vi "Lockin.DAQ.Write AO.vi"(8 "error in (no error)":errorcluster, 10 "AO []":waveform(dbl)[](array[waveform]), 11 "Lockin.DAQ in":refnum<class "Lockin.DAQ.lvclass">) -> (0 "error out":errorcluster, 1 "AO time (ms)":u32=53, 3 "Lockin.DAQ out":refnum<class "Lockin.DAQ.lvclass">)   [LabVIEW 2016, in "Lockin.DAQ.lvclass"]
uses:
  Lockin.DAQ.lvclass
  Lockin.DAQ.lvclass/Lockin.DAQ.ctl
  <vilib>/DAQmx/write.llb/DAQmx Write (Analog 1D Wfm NChan NSamp).vi
  <vilib>/DAQmx/miscellaneous.llb/DAQmx Fill In Error Info.vi
panel:
  out "P Check":bool[](array[boolean])
  out "# samples written":u32[](array[numeric])
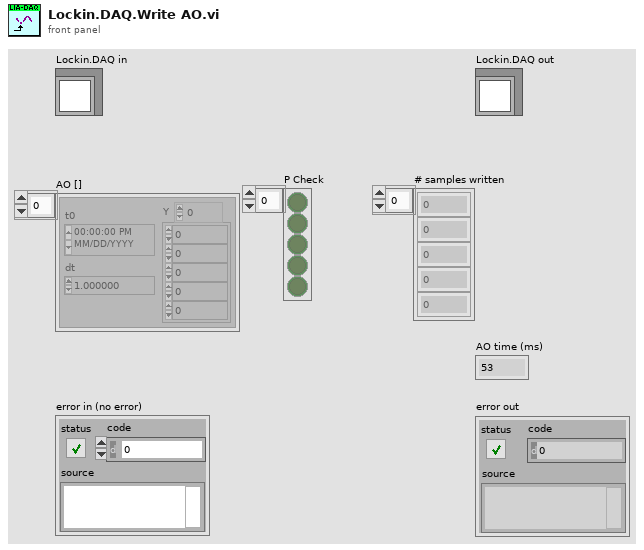
[diagram p1: front panel]
types:
  T1 = enum16{"static", "dynamic", "dynamic asynchronous"}
  T2 = typedef "Lockin.DAQ.lvclass/DAQType-enum.ctl" = enum16{"None", "USB 4431", "PXI 446x"}
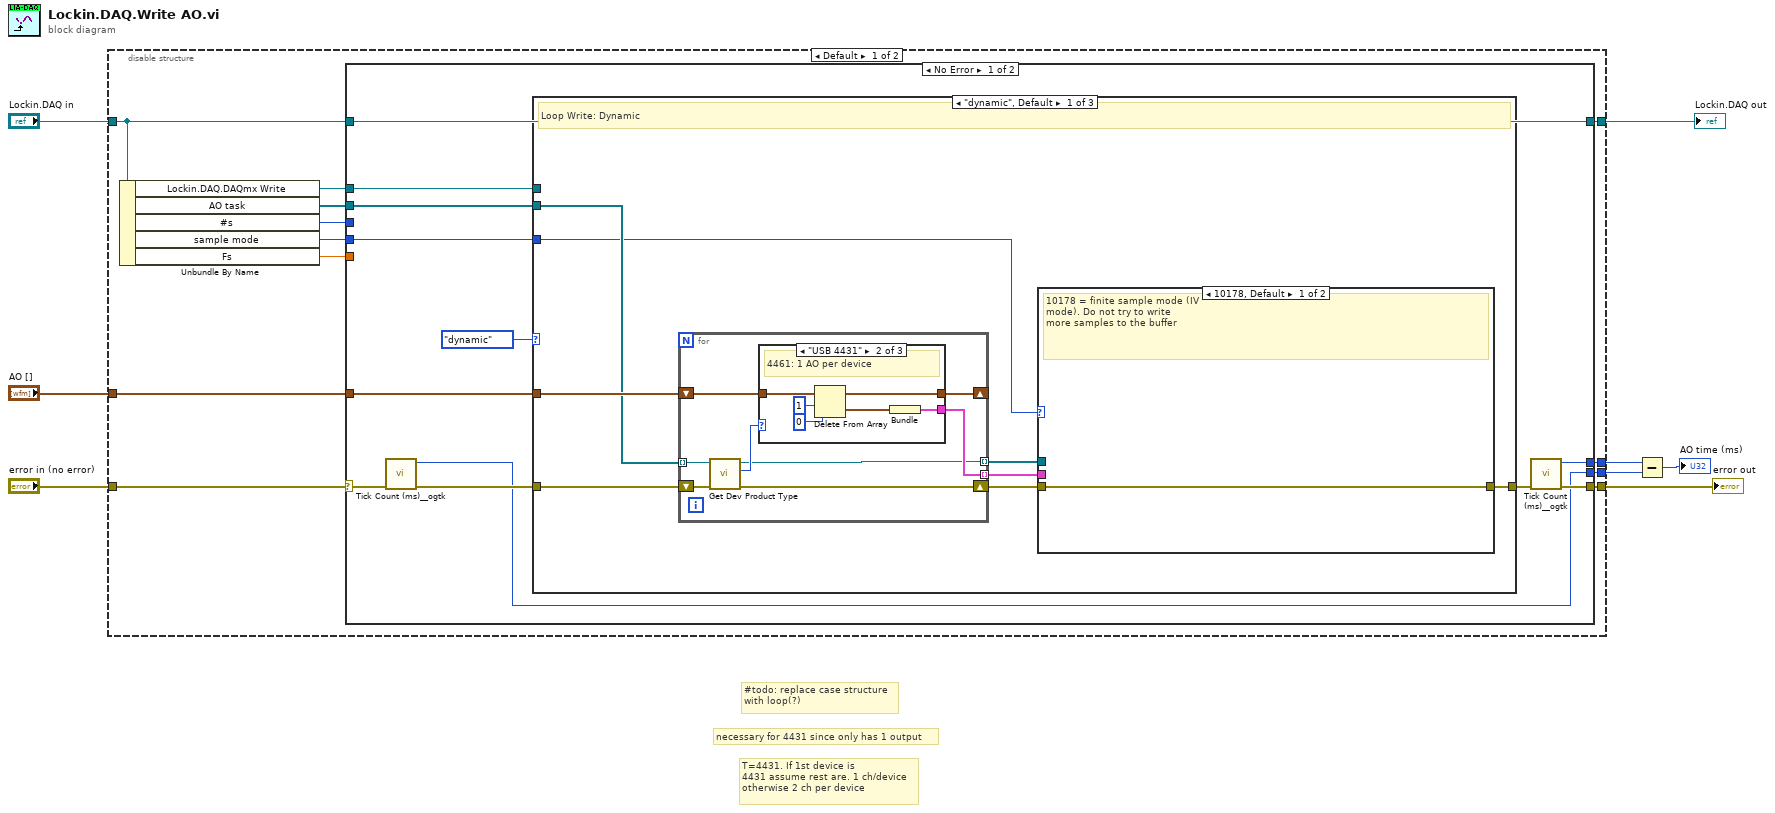
[diagram p0: block diagram]
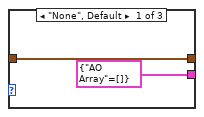
[diagram p2: hidden frame]
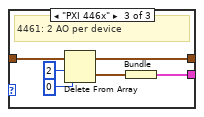
[diagram p3: hidden frame]
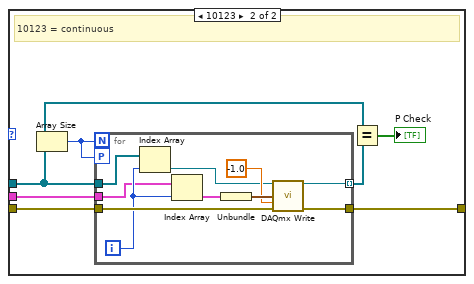
[diagram p4: hidden frame]
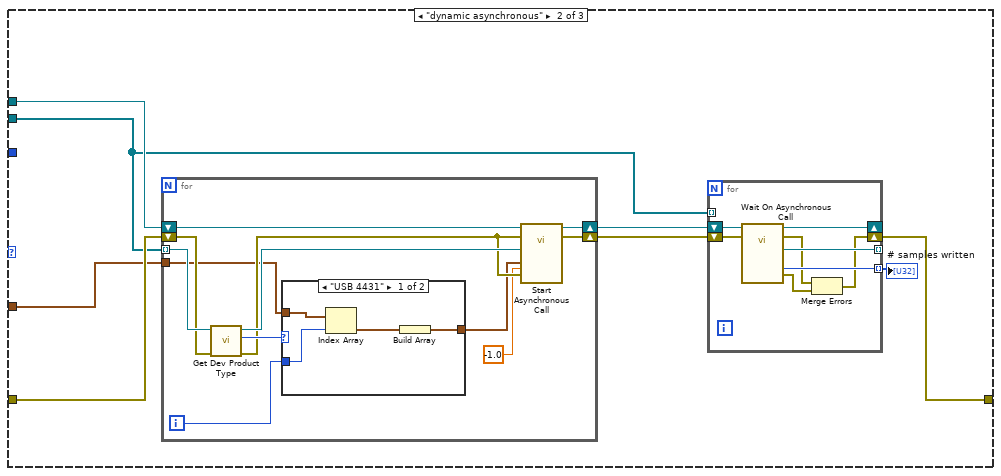
[diagram p5: hidden frame]
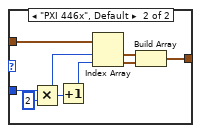
[diagram p6: hidden frame]
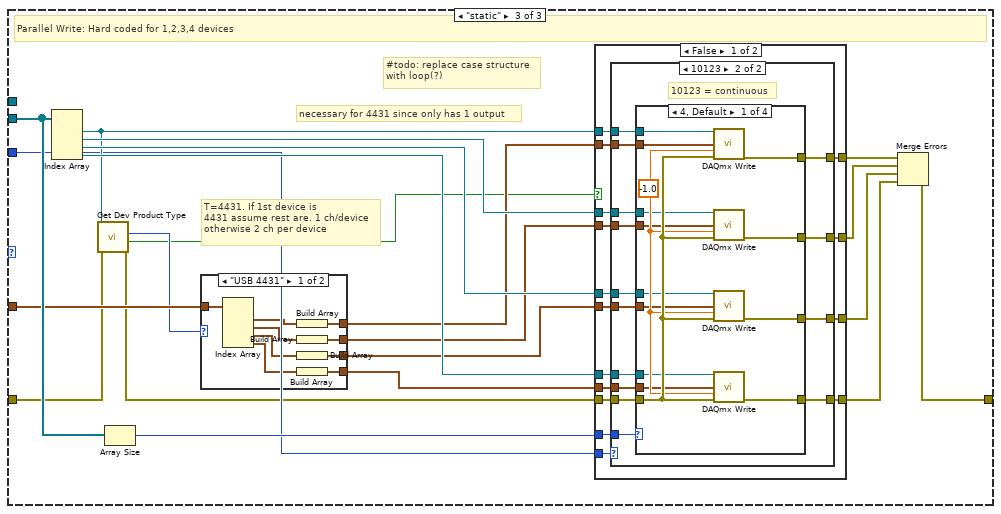
[diagram p7: hidden frame]
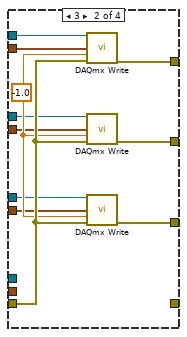
[diagram p9: hidden frame]
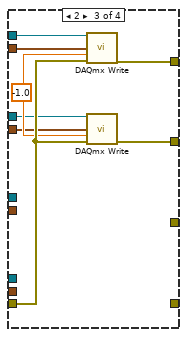
[diagram p10: hidden frame]
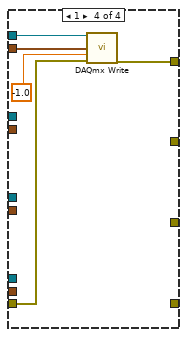
[diagram p11: hidden frame]
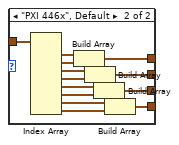
[diagram p13: hidden frame]
diagram:
  # "#todo: replace case structure\nwith loop(?)"
  # "T=4431. If 1st device is \n4431 assume rest are. 1 ch/device\notherwise 2 ch per device"
  # "necessary for 4431 since only has 1 output"
  n1 = disable-structure shown="Default" {
    disable-tunnel: [w18 w236] -> w3
    disable-tunnel: "Lockin.DAQ in" -> [w16 _]
    disable-tunnel: "AO []" -> [w17 w235]
    disable-tunnel: "error in (no error)" -> [w10 w236]
    disable-tunnel: [w15 _] -> w2
    disable-tunnel: [w14 _] -> w7
    disable-tunnel: [w13 _] -> w6
    frame condition #0 (active) {
      n2 = Unbundle By Name(w16) -> ("Lockin.DAQ.DAQmx Write"=w9:refnum<vi>, "AO task"=w11:refnum<k21>[], "#s"=w20:i32, "sample mode"=w19:i32, "Fs"=w12:dbl)
      n3 = case shown="No Error" w10 {
        selector: w10 -> [w25 w233]
        tunnel: w20 -> [_ _]
        tunnel: w19 -> [w26 _]
        tunnel: [w29 w233] -> w18
        tunnel: w17 -> [w31 _]
        tunnel: w11 -> [w32 _]
        tunnel: w16 -> [w27 w234]
        tunnel: [w27 w234] -> w15
        tunnel: [w28 _] -> w14
        tunnel: [w21 _] -> w13
        tunnel: w12 -> [_ _]
        tunnel: w9 -> [w23 _]
        frame No Error {
          n4 = call <userlib>:"Tick Count (ms)__ogtk.vi"("error in (no error)"=w25) -> ("error out"=w24:errorcluster, "millisecond timer value"=w21:u32)  [unwired: 9 in]
          n5 = case shown="\"dynamic\", Default" T1."dynamic" ("Enum") {
            tunnel: w32 -> [w35 w82 w141]
            tunnel: w31 -> [w38 w84 w140]
            tunnel: [w37 w83 w139] -> w30
            tunnel: w26 -> [w33 _ w125]
            tunnel: w24 -> [w40 w86 w123]
            tunnel: w23 -> [_ w85 _]
            frame "dynamic", Default {
              # "Loop Write: Dynamic"
              n6 = for {
                tunnel: [w44] -> w36 mode=indexing
                shift-right: [w47] -> w39
                shift-left: w40 -> [w48]
                tunnel: w35 -> [w43] mode=indexing
                tunnel: [w42] -> w34 mode=indexing
                shift-right: [w41] -> _
                shift-left: w38 -> [w46]
                n7 = call "Get Dev Product Type.vi"("error in (no error)"=w48, "Refnum in"=w43) -> ("error out"=w47:errorcluster, "DAQ Type"=w45:T2, "Refnum out"=w42:refnum<k21>)  [unwired: 6 in, 1 out]
                n8 = case shown="\"USB 4431\"" w45 {
                  tunnel: w46 -> [w50 w56 w62]
                  tunnel: [w50 w55 w61] -> w41
                  tunnel: [cluster{"AO Array":waveform(dbl)[]} {"AO Array"=[]} w53 w58] -> w44
                  frame "None", Default {
                  }
                  frame "USB 4431" {
                    # "4461: 1 AO per device"
                    n9 = Delete From Array(array=w56, length=1, index=0) -> (deleted portion=w52:waveform(dbl)[], array with subset deleted=w55:waveform(dbl)[])
                    n10 = Bundle("AO []"=w52) -> (w53:cluster{"AO []":waveform(dbl)[]})  [unwired: 1 in]
                  }
                  frame "PXI 446x" {
                    # "4461: 2 AO per device"
                    n11 = Delete From Array(array=w62, length=2, index=0) -> (deleted portion=w59:waveform(dbl)[], array with subset deleted=w61:waveform(dbl)[])
                    n12 = Bundle("AO []"=w59) -> (w58:cluster{"AO []":waveform(dbl)[]})  [unwired: 1 in]
                  }
                }
              }
              n13 = case shown="10178, Default" w33 {
                tunnel: [w63 w68] -> w37
                tunnel: w34 -> [_ w65]
                tunnel: w36 -> [_ w70]
                tunnel: w39 -> [w63 w69]
                frame 10178, Default {
                  # "10178 = finite sample mode (IV\nmode). Do not try to write\nmore samples to the buffer"
                }
                frame 10123 {
                  # "10123 = continuous"
                  n14 = Array Size(array=w65) -> (size(s)=w67:i32)
                  n15 = for {
                    N: w67 -> [_]
                    tunnel: w65 -> [w71]
                    tunnel: w70 -> [w72]
                    tunnel: w69 -> [w80]
                    tunnel: [w79] -> w68
                    workers-P: w67 -> [_]
                    tunnel: [w76] -> w66 mode=indexing
                    i -> [w73]
                    n16 = Index Array(array=w71, index=w73) -> (element=w74:refnum<k21>)
                    n17 = Index Array(array=w72, index=w73) -> (element=w75:cluster{"AO []":waveform(dbl)[]})
                    n18 = Unbundle(w75) -> ("AO []"=w78:waveform(dbl)[])
                    n19 = call-poly <vilib>:"DAQmx Write.vi"("task/channels in"=w74, "data"=w78, "timeout"=-1.0, "error in"=w80) -> ("task out"=w76:refnum<k21>, "error out"=w79:errorcluster)  [unwired: 9 in, 1 out]
                  }
                  n20 = Equal?(x=w65, y=w66) -> (x = y?=→"P Check":bool[])
                }
              }
            }
            frame "dynamic asynchronous" {
              n21 = for {
                shift-right: [w100] -> w87
                shift-left: w86 -> [w94]
                shift-right: [w99] -> w88
                shift-left: w85 -> [w98]
                tunnel: w82 -> [w96] mode=indexing
                tunnel: w84 -> [w92]
                i -> [w91]
                n22 = call "Get Dev Product Type.vi"("error in (no error)"=w94, "Refnum in"=w96) -> ("error out"=w93:errorcluster, "DAQ Type"=w97:T2, "Refnum out"=w95:refnum<k21>)  [unwired: 6 in, 1 out]
                n23 = case shown="\"USB 4431\"" w97 {
                  tunnel: [w103 w110] -> w90
                  tunnel: w92 -> [w102 w109]
                  tunnel: w91 -> [w101 w107]
                  frame "USB 4431" {
                    n24 = Index Array(array=w102, index=w101) -> (element=w104:waveform(dbl))
                    n25 = Build Array(w104) -> (w103:waveform(dbl)[])
                  }
                  frame "PXI 446x", Default {
                    n26 = Multiply(x=w107, y=2) -> (x*y=w106:i32)
                    n27 = Increment(x=w106) -> (x+1=w105:i32)
                    n28 = Index Array(array=w109, index #1=w106, index #2=w105) -> (element #1=w111:waveform(dbl), element #2=w112:waveform(dbl))
                    n29 = Build Array(w111, w112) -> (w110:waveform(dbl)[])
                  }
                }
                n30 = call-by-ref "Start Asynchronous Call"(reference=w98, error in=w93, "Refnum in"=w95, "data"=w90, "timeout"=-1.0, 11:"error in (no error)"=w93) -> (reference out=w99:refnum<vi>, error out=w100:errorcluster)  [unwired: 8 in, 4 out]
              }
              n31 = for {
                shift-right: [w113] -> w83
                shift-left: w87 -> [w119]
                shift-right: [w118] -> _
                shift-left: w88 -> [w120]
                tunnel: [w117] -> _ mode=indexing
                tunnel: [w116] -> w81 mode=indexing
                tunnel: w82 -> [_] mode=indexing
                n32 = call-by-ref "Wait On Asynchronous Call"(reference=w120, error in=w119) -> (reference out=w118:refnum<vi>, error out=w114:errorcluster, "Refnum out"=w117:refnum<k21>, "number of samples written per channel"=w116:u32, 15:"error out"=w115:errorcluster)  [unwired: 12 in, 1 out]
                n33 = Merge Errors(w114, w115) -> (w113:errorcluster)
              }
              "# samples written" <- w81
            }
            frame "static" {
              # "#todo: replace case structure\nwith loop(?)"
              # "T=4431. If 1st device is \n4431 assume rest are. 1 ch/device\notherwise 2 ch per device"
              # "necessary for 4431 since only has 1 output"
              # "Parallel Write: Hard coded for 1,2,3,4 devices"
              n34 = Index Array(array=w141) -> (element #1=w134:refnum<k21>, element #2=w138:refnum<k21>, element #3=w137:refnum<k21>, element #4=w136:refnum<k21>)  [unwired: 4 in]
              n35 = call "Get Dev Product Type.vi"("error in (no error)"=w123, "Refnum in"=w134) -> ("error out"=w122:errorcluster, "DevIsSimulated"=w124:bool, "DAQ Type"=w130:T2)  [unwired: 6 in, 1 out]
              n36 = Array Size(array=w141) -> (size(s)=w135:i32)
              n37 = case shown="\"USB 4431\"" w130 {
                tunnel: [w219 w225] -> w132
                tunnel: [w218 w224] -> w133
                tunnel: [w217 w223] -> w121
                tunnel: [w215 w221] -> w131
                tunnel: w140 -> [w214 w220]
                frame "USB 4431" {
                  n38 = Index Array(array=w214) -> (element #1=w216:waveform(dbl), element #2=w213:waveform(dbl), element #3=w212:waveform(dbl), element #4=w211:waveform(dbl))  [unwired: 4 in]
                  n39 = Build Array(w216) -> (w215:waveform(dbl)[])
                  n40 = Build Array(w213) -> (w219:waveform(dbl)[])
                  n41 = Build Array(w212) -> (w218:waveform(dbl)[])
                  n42 = Build Array(w211) -> (w217:waveform(dbl)[])
                }
                frame "PXI 446x", Default {
                  n43 = Index Array(array=w220) -> (element #1=w222:waveform(dbl), element #2=w232:waveform(dbl), element #3=w231:waveform(dbl), element #4=w230:waveform(dbl), element #5=w229:waveform(dbl), element #6=w228:waveform(dbl), element #7=w227:waveform(dbl), element #8=w226:waveform(dbl))  [unwired: 8 in]
                  n44 = Build Array(w222, w232) -> (w221:waveform(dbl)[])
                  n45 = Build Array(w231, w230) -> (w225:waveform(dbl)[])
                  n46 = Build Array(w229, w228) -> (w224:waveform(dbl)[])
                  n47 = Build Array(w227, w226) -> (w223:waveform(dbl)[])
                }
              }
              n48 = case shown="False" w124 {
                tunnel: w138 -> [w156 _]
                tunnel: w137 -> [w155 _]
                tunnel: w136 -> [w154 _]
                tunnel: w135 -> [w153 _]
                tunnel: w134 -> [w152 _]
                tunnel: w121 -> [w151 _]
                tunnel: w133 -> [w150 _]
                tunnel: w132 -> [w149 _]
                tunnel: w131 -> [w148 _]
                tunnel: w122 -> [w147 w210]
                tunnel: [w146 _] -> w129
                tunnel: [w145 _] -> w128
                tunnel: [w144 w210] -> w127
                tunnel: [w142 _] -> w126
                tunnel: w125 -> [w143 _]
                frame False {
                  n49 = case shown="10123" w143 {
                    tunnel: w156 -> [_ w171]
                    tunnel: w155 -> [_ w170]
                    tunnel: w154 -> [_ w169]
                    tunnel: [w157 w168] -> w144
                    tunnel: [_ w167] -> w145
                    tunnel: [_ w166] -> w146
                    tunnel: [_ w165] -> w142
                    tunnel: w153 -> [_ w164]
                    tunnel: w152 -> [_ w163]
                    tunnel: w151 -> [_ w162]
                    tunnel: w150 -> [_ w161]
                    tunnel: w149 -> [_ w160]
                    tunnel: w148 -> [_ w159]
                    tunnel: w147 -> [w157 w158]
                    frame 10178, Default {
                      # "10178 = finite sample mode (IV\nmode). Do not try to write\nmore samples to the buffer"
                    }
                    frame 10123 {
                      # "10123 = continuous"
                      n50 = case shown="4, Default" w164 {
                        tunnel: w158 -> [w185 w196 w204 w209]
                        tunnel: w171 -> [w183 w194 w202 _]
                        tunnel: w170 -> [w182 w193 _ _]
                        tunnel: w169 -> [w181 _ _ _]
                        tunnel: w160 -> [w180 w192 w201 _]
                        tunnel: w161 -> [w179 w191 _ _]
                        tunnel: w162 -> [w178 _ _ _]
                        tunnel: [w177 w190 w200 w207] -> w168
                        tunnel: [w176 w189 w199 _] -> w167
                        tunnel: [w175 w188 _ _] -> w166
                        tunnel: [w174 _ _ _] -> w165
                        tunnel: w163 -> [w173 w187 w198 w206]
                        tunnel: w159 -> [w172 w186 w197 w205]
                        frame 4, Default {
                          w184 = -1.0 ("timeout")
                          n51 = call-poly <vilib>:"DAQmx Write.vi"("task/channels in"=w173, "data"=w172, "timeout"=w184, "error in"=w185) -> ("error out"=w177:errorcluster)  [unwired: 9 in, 2 out]
                          n52 = call-poly <vilib>:"DAQmx Write.vi"("task/channels in"=w183, "data"=w180, "timeout"=w184, "error in"=w185) -> ("error out"=w176:errorcluster)  [unwired: 9 in, 2 out]
                          n53 = call-poly <vilib>:"DAQmx Write.vi"("task/channels in"=w182, "data"=w179, "timeout"=w184, "error in"=w185) -> ("error out"=w175:errorcluster)  [unwired: 9 in, 2 out]
                          n54 = call-poly <vilib>:"DAQmx Write.vi"("task/channels in"=w181, "data"=w178, "timeout"=w184, "error in"=w185) -> ("error out"=w174:errorcluster)  [unwired: 9 in, 2 out]
                        }
                        frame 3 {
                          w195 = -1.0 ("timeout")
                          n55 = call-poly <vilib>:"DAQmx Write.vi"("task/channels in"=w187, "data"=w186, "timeout"=w195, "error in"=w196) -> ("error out"=w190:errorcluster)  [unwired: 9 in, 2 out]
                          n56 = call-poly <vilib>:"DAQmx Write.vi"("task/channels in"=w194, "data"=w192, "timeout"=w195, "error in"=w196) -> ("error out"=w189:errorcluster)  [unwired: 9 in, 2 out]
                          n57 = call-poly <vilib>:"DAQmx Write.vi"("task/channels in"=w193, "data"=w191, "timeout"=w195, "error in"=w196) -> ("error out"=w188:errorcluster)  [unwired: 9 in, 2 out]
                        }
                        frame 2 {
                          w203 = -1.0 ("timeout")
                          n58 = call-poly <vilib>:"DAQmx Write.vi"("task/channels in"=w198, "data"=w197, "timeout"=w203, "error in"=w204) -> ("error out"=w200:errorcluster)  [unwired: 9 in, 2 out]
                          n59 = call-poly <vilib>:"DAQmx Write.vi"("task/channels in"=w202, "data"=w201, "timeout"=w203, "error in"=w204) -> ("error out"=w199:errorcluster)  [unwired: 9 in, 2 out]
                        }
                        frame 1 {
                          n60 = call-poly <vilib>:"DAQmx Write.vi"("task/channels in"=w206, "data"=w205, "timeout"=-1.0, "error in"=w209) -> ("error out"=w207:errorcluster)  [unwired: 9 in, 2 out]
                        }
                      }
                    }
                  }
                }
                frame True {
                }
              }
              n61 = Merge Errors(w127, w128, w129, w126) -> (w139:errorcluster)
            }
          }
          n62 = call <userlib>:"Tick Count (ms)__ogtk.vi"("error in (no error)"=w30) -> ("error out"=w29:errorcluster, "millisecond timer value"=w28:u32)  [unwired: 9 in]
        }
        frame Error {
        }
      }
    }
    frame condition #1 {
    }
  }
  "error out" <- w3
  "Lockin.DAQ out" <- w2
  n63 = Subtract(x=w7, y=w6) -> (x-y=→"AO time (ms)":u32)
